vi "Get Drag Over Step Position.vi"(10 "Mouse Interaction Tag":string, 11 "Drag-Drop State in":T1) -> (2 "New Position":i32, 3 "Drag-Drop State out":T1)   [LabVIEW 2020, in "Output Sequencer.lvlib" / "Settings UI.lvclass"]
uses:
  Settings UI.lvclass
  Types/Drag-Drop State.ctl
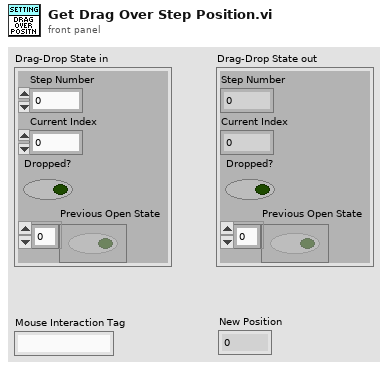
[diagram p1: front panel]
types:
  T1 = typedef "Output Sequencer.lvlib/Settings UI.lvclass/Drag-Drop State.ctl" = cluster{"Step Number":i32, "Current Index":i32, "Dropped?":bool, "Previous Open State":bool[]}
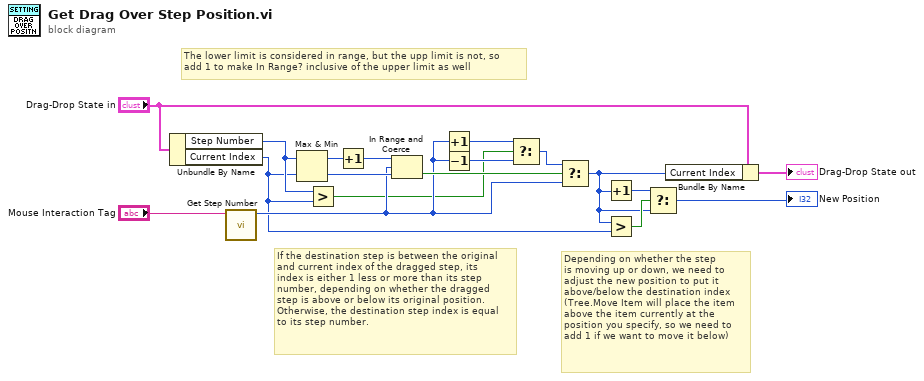
[diagram p0: block diagram]
diagram:
  # "Depending on whether the step\nis moving up or down, we need to\nadjust the new position to put it\nabove/below the destination index\n(Tree.Move Item will place the item\nabove the item currently at the \nposition you specify, so we need to\nadd 1 if we want to move it below)"
  # "If the destination step is between the original\nand current index of the dragged step, its\nindex is either 1 less or more than its step\nnumber, depending on whether the dragged\nstep is above or below its original position.\nOtherwise, the destination step index is equal\nto its step number."
  # "The lower limit is considered in range, but the upp limit is not, so\nadd 1 to make In Range? inclusive of the upper limit as well"
  n1 = Unbundle By Name("Drag-Drop State in") -> ("Step Number"=w8:i32, "Current Index"=w4:i32)
  n2 = call "Get Step Number.vi"("Tree Tag"="Mouse Interaction Tag") -> ("Step Number"=w10:i32)  [unwired: 8 in, 2 out]
  n3 = Max & Min(x=w8, y=w4) -> (max(x,y)=w16:i32, min(x,y)=w17:i32)
  n4 = Greater?(x=w8, y=w4) -> (0:w9:bool)
  n5 = Increment(x=w16) -> (x+1=w15:i32)
  n6 = In Range and Coerce(upper limit=w15, x=w10, lower limit=w17) -> (In Range?=w14:bool)  [unwired: 1 out]
  n7 = Increment(x=w10) -> (x+1=w13:i32)
  n8 = Decrement(x=w10) -> (x-1=w12:i32)
  n9 = Select(t=w13, s=w9, f=w12) -> (s? t:f=w11:i32)
  n10 = Select(t=w11, s=w14, f=w10) -> (s? t:f=w2:i32)
  n11 = Increment(x=w2) -> (x+1=w6:i32)
  n12 = Greater?(x=w2, y=w4) -> (0:w7:bool)
  n13 = Select(t=w6, s=w7, f=w2) -> (s? t:f=→"New Position":i32)
  n14 = Bundle By Name(cluster="Drag-Drop State in", "Current Index"=w2) -> (→"Drag-Drop State out":T1)
